vi "Get Number of Readings in the Buffer.vi"(0 "VISA resource name":refnum<visa-resource-name>, 5 "Timeout (10000 ms)":i32=10000 format="%#.6g", 7 "Buffer Name (defbuffer1)":string="defbuffer1", 11 "error in (no error)":errorcluster) -> (4 "VISA resource name out":refnum<visa-resource-name>, 6 "Data out":string, 15 "error out":errorcluster)   [LabVIEW 2015, in "Keithley 2450.lvlib"]
doc: "This gets the number of readings in the specified buffer"
uses:
  <instrlib>/Keithley 2450/Keithley 2450.lvlib
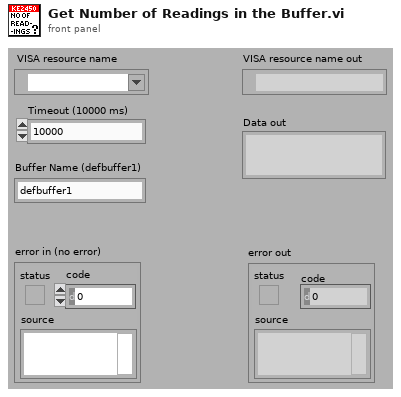
[diagram p1: front panel]
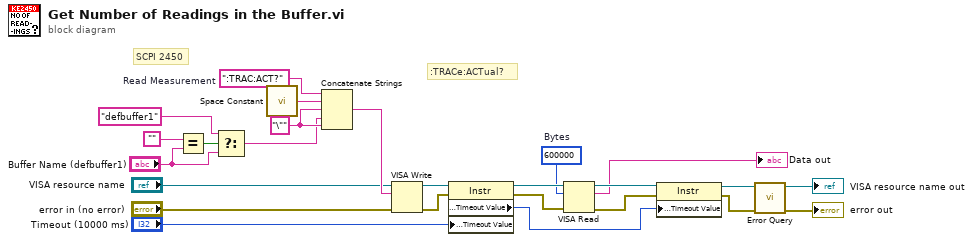
[diagram p0: block diagram]
diagram:
  w10 = "\""
  w7 = ":TRAC:ACT?"  # Read Measurement
  w17 = u32 600000  # Bytes
  # ":TRACe:ACTual?"
  # "SCPI 2450"
  n1 = Equal?(x="", y="Buffer Name (defbuffer1)") -> (x = y?=w13:bool)
  n2 = Select(t="defbuffer1", s=w13, f="Buffer Name (defbuffer1)") -> (s? t:f=w9:string)
  n3 = call <vilib>:"Space Constant.vi"() -> ("String"=w8:string)
  n4 = Concatenate Strings(w7, w8, w10, w9, w10) -> (w24:string)
  n5 = VISA Write(VISA resource name="VISA resource name", write buffer=w24, error in (no error)="error in (no error)") -> (VISA resource name out=w15:refnum<visa-resource-name>, error out=w23:errorcluster)  [unwired: 1 out]
  n6 = property class="Instr"(reference=w15, error in=w23, "General Settings:Timeout Value"="Timeout (10000 ms)") -> (reference out=w22:refnum<visa-resource-name>, error out=w21:errorcluster, "General Settings:Timeout Value"=w18:u32)
  n7 = VISA Read(VISA resource name=w22, byte count=w17, error in (no error)=w21) -> (VISA resource name out=w20:refnum<visa-resource-name>, read buffer=→"Data out":string, error out=w19:errorcluster)  [unwired: 1 out]
  n8 = property class="Instr"(reference=w20, error in=w19, "General Settings:Timeout Value"=w18) -> (reference out=w2:refnum<visa-resource-name>, error out=w1:errorcluster)
  n9 = call <instrlib>:"Error Query.vi"("error in (no error)"=w1, "VISA resource name"=w2) -> ("error out"=→"error out":errorcluster, "VISA resource name out"=→"VISA resource name out":refnum<visa-resource-name>)  [unwired: 8 out]
